vi "uid.set.vi"(8 "error in (no error)":errorcluster, 10 "uid":string, 11 "midi-file-events in":refnum<class "midi-file-event.lvclass">) -> (0 "error out":errorcluster, 3 "midi-file-events out":refnum<class "midi-file-event.lvclass">)   [LabVIEW 2020, in "midi-file-event.lvclass"]
uses:
  midi-file-event.lvclass
  midi-file-event.lvclass/midi-file-event.ctl
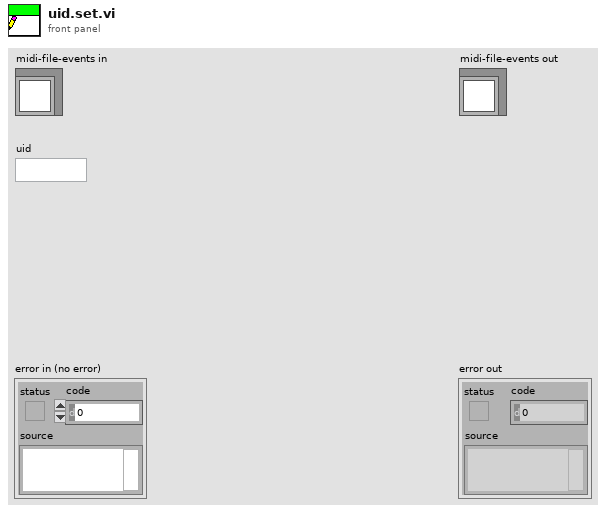
[diagram p1: front panel]
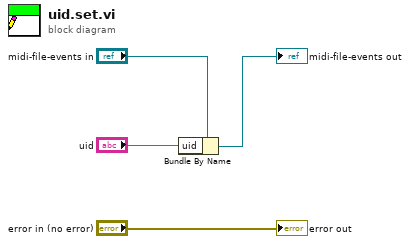
[diagram p0: block diagram]
diagram:
  n1 = Bundle By Name(cluster="midi-file-events in", "uid"="uid") -> (→"midi-file-events out":refnum<class "midi-file-event.lvclass">)
  "error out" <- "error in (no error)"
